vi "WaitForACK.vi"   [LabVIEW 2020]
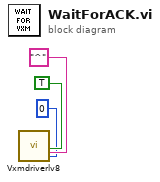
[diagram p0: block diagram]
diagram:
  n1 = call "Vxmdriverlv8.Vi"("Wait\nfor \nchar"=TRUE, "Char(s) to wait for"="^", "Char\nTimeout\nTime (ms)"=0) -> ()  [unwired: 19 in, 6 out]
